vi "ziExample-Boxcar.vi"() -> ()   [LabVIEW 2009]
doc: "Control a Zurich instrument device via the LabOne Labview API. \nRequirements: Zurich Instruments UHFLI \nThis example retrives boxcar samples from a Zurich Instruments UHFLI instrument.\n\n© Zurich Instruments AG, www.zhinst.com"
uses:
  <instrlib>/Zurich Instruments LabOne/Public/Configure/ziSetValueDoubleArray.vi
  <instrlib>/Zurich Instruments LabOne/Public/Utility/ziTicksToS_vector.vi
  <instrlib>/Zurich Instruments LabOne/Public/Data/ziGetEventDoubleDataTS.vi
  <instrlib>/Zurich Instruments LabOne/Public/Utility/ziTicksToS_single.vi
  <instrlib>/Zurich Instruments LabOne/Zurich Instruments LabOne.lvlib
panel:
  out "Error Out":errorcluster
  out "Sample Rate (1/s)":cluster{"Timestamp(s)":dbl[], "Value":dbl[]}(graph)
  in  "Address":string="DEV"
  out "Selected Device":string
  out "Update Rate (1/s)":dbl(graph)
  out "All Values (V)":cluster{"Timestamp(s)":dbl[], "Value":dbl[]}(graph)
  out "Single Values":dbl format="%#_6p"
  in  "stop":bool
  # "ziExample-Boxcar.vi\nRequirements: UHFLI\nsee block diagram for VI description"
  # "Tested Devices:\n- UHFLI"
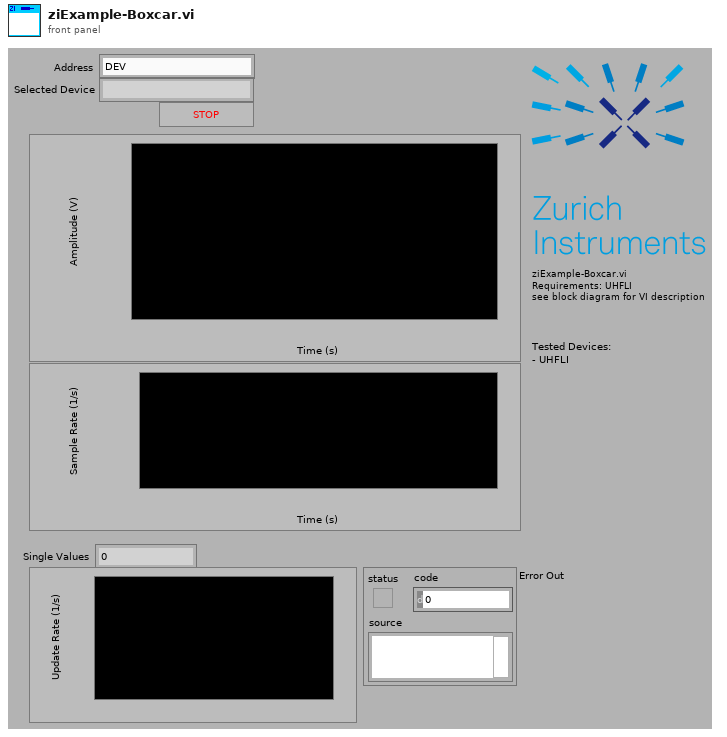
[diagram p1: front panel]
types:
  T1 = typedef "Zurich Instruments LabOne.lvlib/ziTypeHandle.ctl" = cluster{"handleValid":bool, "Conn":u64, "Path Prefix":string, "Handle":u64, "Connected":bool, "Clockbase(s)":dbl}
  T2 = typedef "Zurich Instruments LabOne.lvlib/ziTypeDoubleDataTS.ctl" = cluster{"Timestamp (ticks)":u64[], "Value":dbl[]}
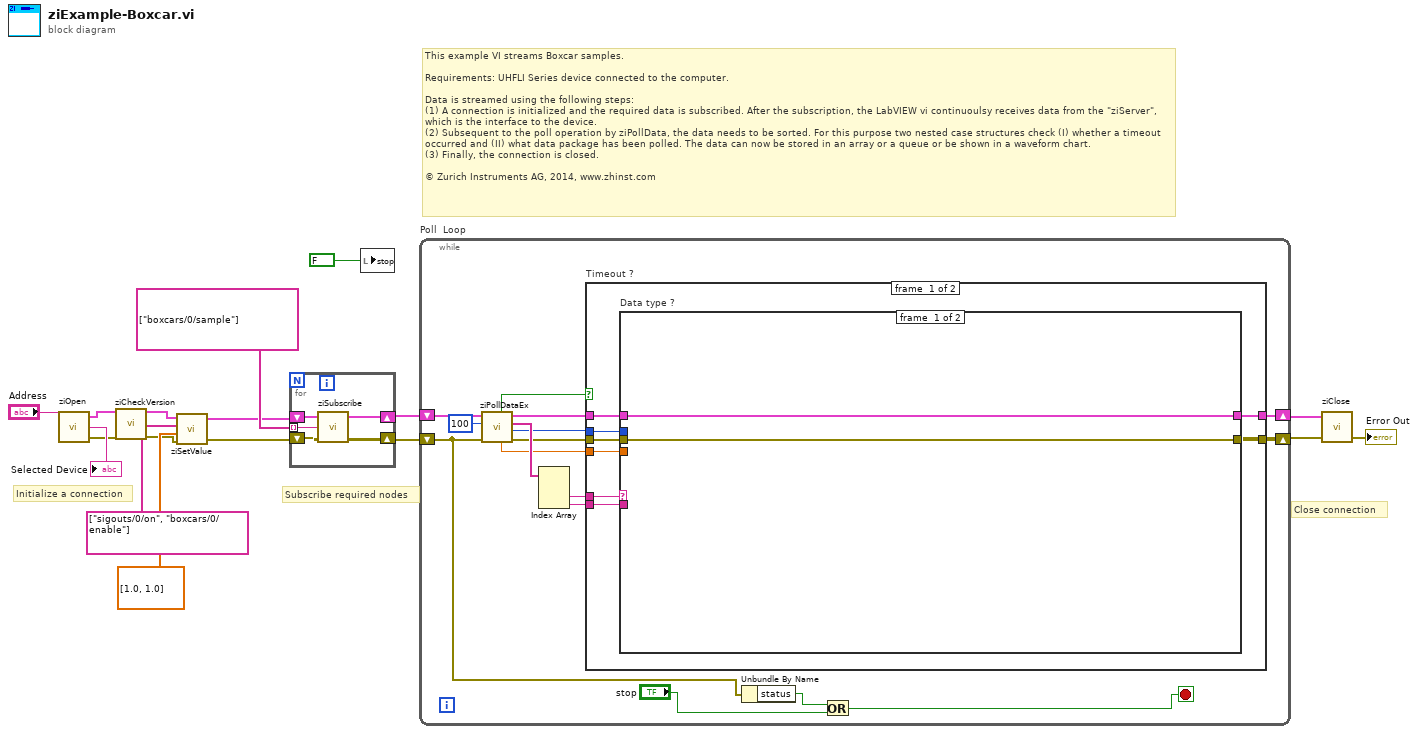
[diagram p0: block diagram]
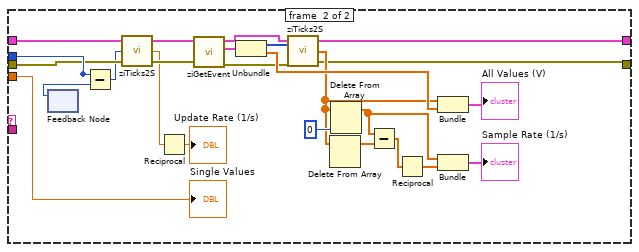
[diagram p2: hidden frame]
diagram:
  # "Close connection"
  # "Initialize a connection"
  # "Subscribe required nodes"
  # "This example VI streams Boxcar samples.\n\nRequirements: UHFLI Series device connected to the computer.\n\nData is streamed using the following steps:\n(1) A connection is initialized and the required data is subscribed. After the subscription, the LabVIEW vi continuoulsy receives data from the \"ziServer\", which is the interface to the device. \n(2) Subsequent to the poll operation by ziPollData, the data needs to be sorted. For this purpose two nested case structures check (I) whether a timeout occurred and (II) what data package has been polled. The data can now be stored in an array or a queue or be shown in a waveform chart. \n(3) Finally, the connection is closed. \n\n© Zurich Instruments AG, 2014, www.zhinst.com"
  n1 = call <instrlib>:"ziOpen.vi"("Address"="Address") -> ("Error Out"=w1:errorcluster, "Selected Device"=→"Selected Device":string, "HandleOut"=w4:T1)  [unwired: 1 in, 2 out]
  n2 = call <instrlib>:"ziCheckVersion.vi"("Handle In"=w4, "Error In"=w1) -> ("Handle Out"=w3:T1, "Error Out"=w2:errorcluster)  [unwired: 11 in, 1 out]
  n3 = call-poly <instrlib>:"ziSetValue.vi"("Error In"=w2, "Values"=dbl[] [1.0, 1.0], "Paths"=string[] ["sigouts/0/on", "boxcars/0/enable"], "Handle In"=w3) -> ("Error Out"=w7:errorcluster, "Handle Out"=w6:T1)  [unwired: 1 in]
  n4 = for {
    shift-right: [w22] -> w13
    shift-left: w6 -> [w20]
    shift-right: [w21] -> w12
    shift-left: w7 -> [w19]
    tunnel: string[] ["boxcars/0/sample"] -> [w18] mode=indexing
    n5 = call <instrlib>:"ziSubscribe.vi"("error in"=w19, "Path ()"=w18, "Handle In"=w20) -> ("error out"=w21:errorcluster, "Handle Out"=w22:T1)  [unwired: 1 in]
  }
  n6 = local write "stop"(FALSE ("Record")) -> ()
  n7 = while "Poll  Loop" {
    shift-right: [w31] -> w14
    shift-left: w13 -> [w38]
    shift-right: [w29] -> w15
    shift-left: w12 -> [w25]
    stop <- w23 stop-if-true
    n8 = call <instrlib>:"ziPollDataEx.vi"("error in"=w25, "Timeout ms (50)"=100 ("TimeOut ms (50)"), "Handle In"=w38) -> ("error out"=w30:errorcluster, "Timestamp (ticks)"=w33:u64, "PathArray"=w35:string[], "Handle Out"=w32:T1, "Value Double"=w28:dbl, "Timed Out"=w36:bool)  [unwired: 1 in, 2 out]
    n9 = Index Array(array=w35) -> (element #2=w34:string, element #3=w27:string)  [unwired: 3 in, 1 out]
    n10 = case "Timeout ?" shown="False" w36 {
      tunnel: w34 -> [w46 _]
      tunnel: w33 -> [w45 _]
      tunnel: w32 -> [w44 w75]
      tunnel: [w43 w75] -> w31
      tunnel: w30 -> [w42 w74]
      tunnel: [w41 w74] -> w29
      tunnel: w28 -> [w40 _]
      tunnel: w27 -> [w39 _]
      frame #0 {
        n11 = case "Data type ?" shown="\"BOXCARS\"" w46 {
          tunnel: w45 -> [_ w72]
          tunnel: w44 -> [w48 w71]
          tunnel: [w48 w53] -> w43
          tunnel: w42 -> [w47 w70]
          tunnel: [w47 w50] -> w41
          tunnel: w40 -> [_ w73]
          tunnel: w39 -> [_ _]
          frame #0 {
          }
          frame #1 {
            n12 = feedback #1() -> (w67:u64)  [unwired: 1 in]
            n13 = Subtract(x=w72, y=w67) -> (x-y=w66:u64)
            n14 = call-poly <instrlib>:"ziTicks2S.vi"("Error In"=w70, "Timestamp(ticks)"=w66, "Handle In"=w71) -> ("Error Out"=w64:errorcluster, "Timestamp(s)"=w63:dbl, "Handle Out"=w65:T1)
            n15 = Reciprocal(x=w63) -> (1/x=→"Update Rate (1/s)":dbl)
            n16 = call-poly <instrlib>:"ziGetEvent.vi"("Error In"=w64, "Handle In"=w65) -> ("Error Out"=w52:errorcluster, "Sample Out"=w69:T2, "Handle Out"=w51:T1)  [unwired: 7 in]
            n17 = Unbundle(w69) -> ("Timestamp (ticks)"=w56:u64[], "Value"=w57:dbl[])
            n18 = call-poly <instrlib>:"ziTicks2S.vi"("Error In"=w52, "Timestamp (ticks)"=w56, "Handle In"=w51) -> ("Error Out"=w50:errorcluster, "Timestamp(s)"=w54:dbl[], "Handle Out"=w53:T1)
            n19 = Delete From Array(array=w54) -> (array with subset deleted=w62:dbl[])  [unwired: 2 in, 1 out]
            n20 = Delete From Array(array=w54, index=0) -> (array with subset deleted=w49:dbl[])  [unwired: 1 in, 1 out]
            n21 = Subtract(x=w49, y=w62) -> (x-y=w55:dbl[])
            n22 = Reciprocal(x=w55) -> (1/x=w59:dbl[])
            n23 = Bundle("Timestamp(s)"=w54, "Value"=w57) -> (→"All Values (V)":cluster{"Timestamp(s)":dbl[], "Value":dbl[]})  [unwired: 1 in]
            n24 = Bundle("Timestamp(s)"=w49, w59) -> (→"Sample Rate (1/s)":cluster{"Timestamp(s)":dbl[], dbl[]})  [unwired: 1 in]
            "Single Values" <- w73
          }
        }
      }
      frame #1 {
        # "Timeout, no action."
      }
    }
    n25 = Unbundle By Name(w25) -> ("status"=w26:bool)
    n26 = Or(x=w26, y="stop") -> (x .or. y?=w23:bool)
  }
  n27 = call <instrlib>:"ziClose.vi"("Error In"=w15, "Handle In"=w14) -> ("Error Out"=→"Error Out":errorcluster)  [unwired: 3 out]
